vi "Matches.vi"(8 "error in (no error)":errorcluster, 10 "Actual":variant, 11 "String Starts With in":refnum<class "String Starts With.lvclass">) -> (0 "error out":errorcluster, 2 "Result":bool, 3 "String Starts With out":refnum<class "String Starts With.lvclass">)   [LabVIEW 2017, in "Transparent Assertions.lvlib" / "String Starts With.lvclass"]
doc: "Evaluates the constraint for <B>Actual</B>. Returns true if the constraint is met."
uses:
  String Starts With.lvclass
  String Starts With.lvclass/String Starts With.ctl
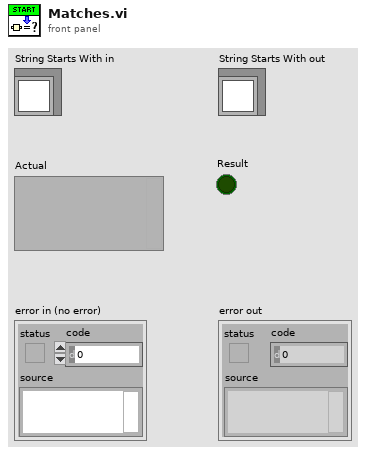
[diagram p1: front panel]
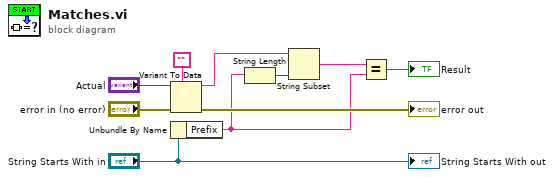
[diagram p0: block diagram]
diagram:
  n1 = Variant To Data(error in="error in (no error)", type="", Variant="Actual") -> (data=w6:string, error out=→"error out":errorcluster)
  n2 = Unbundle By Name("String Starts With in") -> ("Prefix"=w2:string)
  n3 = String Length(string=w2) -> (length=w4:i32)
  n4 = String Subset(string=w6, length (rest)=w4) -> (substring=w3:string)  [unwired: 1 in]
  n5 = Equal?(x=w3, y=w2) -> (x = y?=→"Result":bool)
  "String Starts With out" <- "String Starts With in"
